vi "Drive_Read_Sensors.vi"() -> (3 "Drive Sensor Readings":T1)   [LabVIEW 2012]
uses:
  <vilib>/Rock Robotics/WPI/CAN/Jaguar/SubVIs/WPI_CANJaguar_StatusSelect.ctl
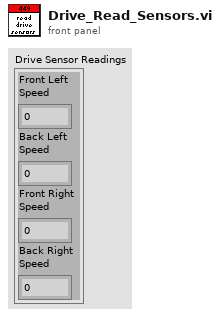
[diagram p1: front panel]
types:
  T1 = cluster{"Front Left\nSpeed":dbl, "Back Left\nSpeed":dbl, "Front Right\nSpeed":dbl, "Back Right\nSpeed":dbl}
  T2 = typedef "WPI_CANJaguar_StatusSelect.ctl" = enum16{"Output Percent VBus", "Output Voltage", "Bus Voltage", "Current", "Temperature", "Position", "Speed", "Limit Switches", "Faults", "Fault Counters", "Power Cycle"}
  T3 = typedef "WPI_MotorControlDeviceRef.ctl" = cluster{"DeviceStatus":errorcluster, "Type":enum16{"PWM", "CAN"}, "PWM":cluster{"Digital Module":T4, "PWM Channel":T5, "DeadBand":T6}, "CAN":cluster{"Device Number":u8, "Control Mode":T7, "Semaphore":T8, "Max Vout":dbl}, "Invert":bool, "TransformRef":T9, "InvTransformRef":T9}
  T4 = typedef "FPGA_TypedefDigitalModule.ctl" = enum16{"Digital Module 1", "Digital Module 2"}
  T5 = typedef "FPGA_DIOPWMChannel.ctl" = enum8{"PWM 1", "PWM 2", "PWM 3", "PWM 4", "PWM 5", "PWM 6", "PWM 7", "PWM 8", "PWM 9", "PWM 10", "Invalid"}
  T6 = typedef "WPI_PWMDeadband.ctl" = cluster{"Name":string, "maxPositivePwm":i32, "minPositivePwm":i32, "centerPwm":i32, "maxNegativePwm":i32, "minNegativePwm":i32, "angularRange":u16}
  T7 = typedef "WPI_CANJaguar_ControlMode.ctl" = enum8{"Percent VBus", "Current", "Speed", "Position", "Voltage"}
  T8 = typedef "Semaphore RefNum" = refnum<k1>
  T9 = typedef "WPI_PWMTransform_ConPane.ctl" = refnum<vi>
  T10 = typedef "WPI_CANJaguar_Status.ctl" = cluster{"Output Percent VBus":dbl, "Output Voltage":dbl, "Bus Voltage":dbl, "Current":dbl, "Temperature":dbl, "Position":dbl, "Speed":dbl, "Limits":cluster{"Forward Limit":bool, "Reverse Limit":bool, "Forward Soft Limit":bool, "Reverse Soft Limit":bool, "Sticky Forward Limit":bool, "Sticky Reverse Limit":bool, "Sticky Forward Soft Limit":bool, "Sticky Reverse Soft Limit":bool}, "Faults":cluster{"Current Fault":bool, "Temperature Fault":bool, "Bus Voltage Fault":bool, "Gate Driver Fault":bool, "Comm Fault":bool}, "Fault Counters":cluster{"Current Faults":u8, "Temperature Faults":u8, "Bus Voltage Faults":u8, "Gate Driver Faults":u8, "Comm Faults":u8, "CAN Status":u8, "CAN RX Errors":u8, "CAN TX Errors":u8}, "Power Cycle":bool}
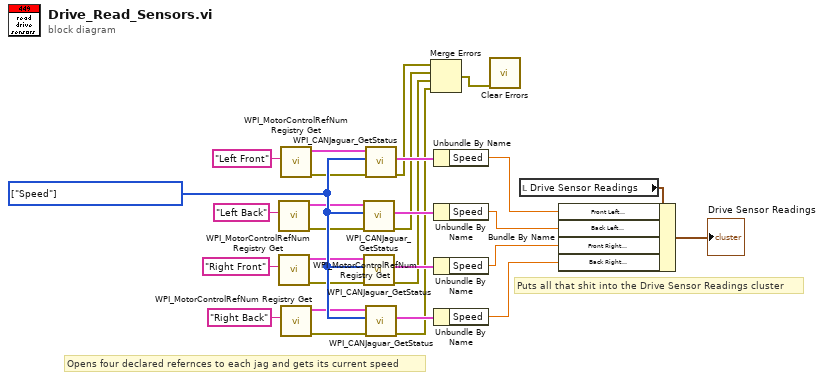
[diagram p0: block diagram]
diagram:
  w24 = T2[] [enum."Speed"] items=["Output Percent VBus", "Output Voltage", "Bus Voltage", "Current", "Temperature", "Position", "Speed", "Limit Switches", "Faults", "Fault Counters", "Power Cycle"] ("Status Select")
  # "Puts all that shit into the Drive Sensor Readings cluster"
  # "Opens four declared refernces to each jag and gets its current speed"
  n1 = call <vilib>:"WPI_MotorControlRefNum Registry Get.vi"("refnum name"="Left Back") -> ("error out"=w12:errorcluster, "MotorControlDevRef"=w7:T3)  [unwired: 9 in]
  n2 = call <vilib>:"WPI_MotorControlRefNum Registry Get.vi"("refnum name"="Right Front") -> ("error out"=w16:errorcluster, "MotorControlDevRef"=w8:T3)  [unwired: 9 in]
  n3 = call <vilib>:"WPI_MotorControlRefNum Registry Get.vi"("refnum name"="Left Front") -> ("error out"=w14:errorcluster, "MotorControlDevRef"=w9:T3)  [unwired: 9 in]
  n4 = call <vilib>:"WPI_MotorControlRefNum Registry Get.vi"("refnum name"="Right Back") -> ("error out"=w10:errorcluster, "MotorControlDevRef"=w6:T3)  [unwired: 9 in]
  n5 = call <vilib>:"WPI_CANJaguar_GetStatus.vi"("error in (no error)"=w12, "Status Select"=w24, "CAN Jaguar Ref"=w7) -> ("error out"=w20:errorcluster, "Status"=w27:T10)  [unwired: 6 in, 1 out]
  n6 = call <vilib>:"WPI_CANJaguar_GetStatus.vi"("error in (no error)"=w16, "Status Select"=w24, "CAN Jaguar Ref"=w8) -> ("error out"=w19:errorcluster, "Status"=w26:T10)  [unwired: 6 in, 1 out]
  n7 = call <vilib>:"WPI_CANJaguar_GetStatus.vi"("error in (no error)"=w14, "Status Select"=w24, "CAN Jaguar Ref"=w9) -> ("error out"=w21:errorcluster, "Status"=w28:T10)  [unwired: 6 in, 1 out]
  n8 = call <vilib>:"WPI_CANJaguar_GetStatus.vi"("error in (no error)"=w10, "Status Select"=w24, "CAN Jaguar Ref"=w6) -> ("error out"=w18:errorcluster, "Status"=w25:T10)  [unwired: 6 in, 1 out]
  n9 = Merge Errors(w21, w20, w19, w18) -> (w1:errorcluster)
  n10 = Unbundle By Name(w28) -> ("Speed"=w23:dbl)
  n11 = Unbundle By Name(w27) -> ("Speed"=w2:dbl)
  n12 = Unbundle By Name(w26) -> ("Speed"=w3:dbl)
  n13 = Unbundle By Name(w25) -> ("Speed"=w22:dbl)
  n14 = call <vilib>:"Clear Errors.vi"("error in (no error)"=w1) -> ()  [unwired: 6 in, 1 out]
  n15 = local read "Drive Sensor Readings"() -> (w4:T1)
  n16 = Bundle By Name(cluster=w4, "Front Left\nSpeed"=w23, "Back Left\nSpeed"=w2, "Front Right\nSpeed"=w3, "Back Right\nSpeed"=w22) -> (→"Drive Sensor Readings":T1)
